vi "Send Move Command.vi"(0 "CS++Motor in":refnum<class "CS++Motor.lvclass">, 1 "Moving?":bool[](array[boolean]), 3 "MovementList In":T1(array[cluster]), 5 "error in (no error)":errorcluster, 6 "Axis Overwrite?":bool, 7 "LastPos In":dbl[](array[numeric]), 8 "SimultaneousMovement?":bool, 11 "ActPos":dbl[](array[numeric])) -> (13 "LastPos Out":dbl[](array[numeric]), 14 "CS++Motor out":refnum<class "CS++Motor.lvclass">, 17 "MovementList Out":T1(array[cluster]), 19 "error out":errorcluster)   [LabVIEW 2015, in "CS++Motor.lvlib" / "CS++Motor.lvclass"]
doc: "This VI sends the Movement Commands to the child class if necessary."
uses:
  CS++Motor.lvclass
  CSPP_Core/Classes/CS++ProcessVariables/ProcessVariable/PV.lvclass
  PV-Enum-n.ctl
  CS++Motor.lvclass/CS++Motor.ctl
  CSPP_Core/Classes/CS++ProcessVariables/ProcessVariable/PV.lvclass/PV.ctl
  CSPP_Core/Classes/CS++ProcessVariables/ProcessVariable/Write Data.vi
  CSPP_Core/Classes/CS++ProcessVariables/ProcessVariable/Write Timestamp.vi
  CSPP_Core/Classes/CS++ProcessVariables/ProcessVariable/Write Quality.vi
  CSPP_Core/Classes/CS++ProcessVariables/ProcessVariable/Write status.vi
  CSPP_Core/Classes/CS++ProcessVariables/PVConnection/PVConnection.lvclass
  CSPP_Core/Libraries/Utilities/CS++Utilities.lvlib
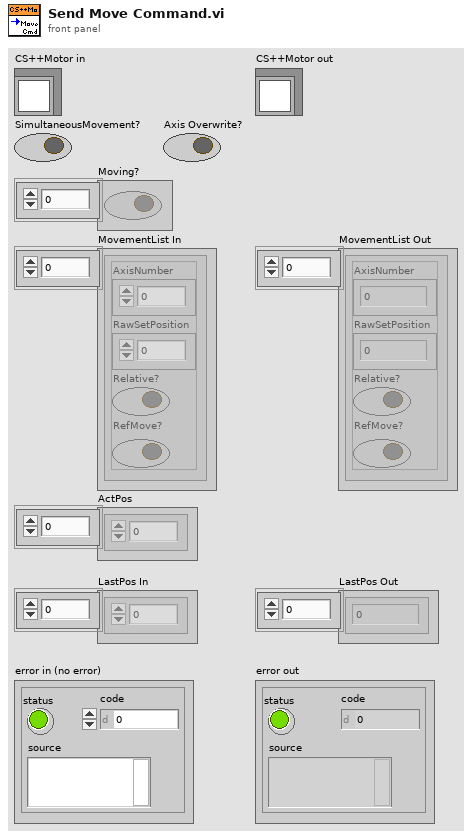
[diagram p1: front panel]
types:
  T1 = cluster{"AxisNumber":u8, "RawSetPosition":dbl, "Relative?":bool, "RefMove?":bool}[]
  T2 = typedef "CS++Motor.lvlib/CS++Motor.lvclass/PV-Enum-n.ctl" = enum16{"PhysicalName", "unit", "ActPosition", "SetPosition", "RawSetPosition", "StartVelocity", "StopVelocity", "Acceleration", "RangeMin", "RangeMax", "Scaling", "RangeRefError", "LogicalPositionArray", "NoOfCommands"}
  T3 = cluster{"AxisNumber":u8, "RawSetPosition":dbl, "Relative?":bool, "RefMove?":bool}
  T4 = cluster{"LogicalName":string, "PhysicalName":string, "unit":string, "Scaling":dbl, "StartVelocity":dbl, "StopVelocity":dbl, "Acceleration":dbl, "RangeMin":dbl, "RangeMax":dbl, "LogicalPos-Array":cluster{"LogicalPosition":string, "SetPosition":dbl}[]}[]
  T5 = cluster{"LogicalName":string, "PhysicalName":string, "unit":string, "Scaling":dbl, "StartVelocity":dbl, "StopVelocity":dbl, "Acceleration":dbl, "RangeMin":dbl, "RangeMax":dbl, "LogicalPos-Array":cluster{"LogicalPosition":string, "SetPosition":dbl}[]}
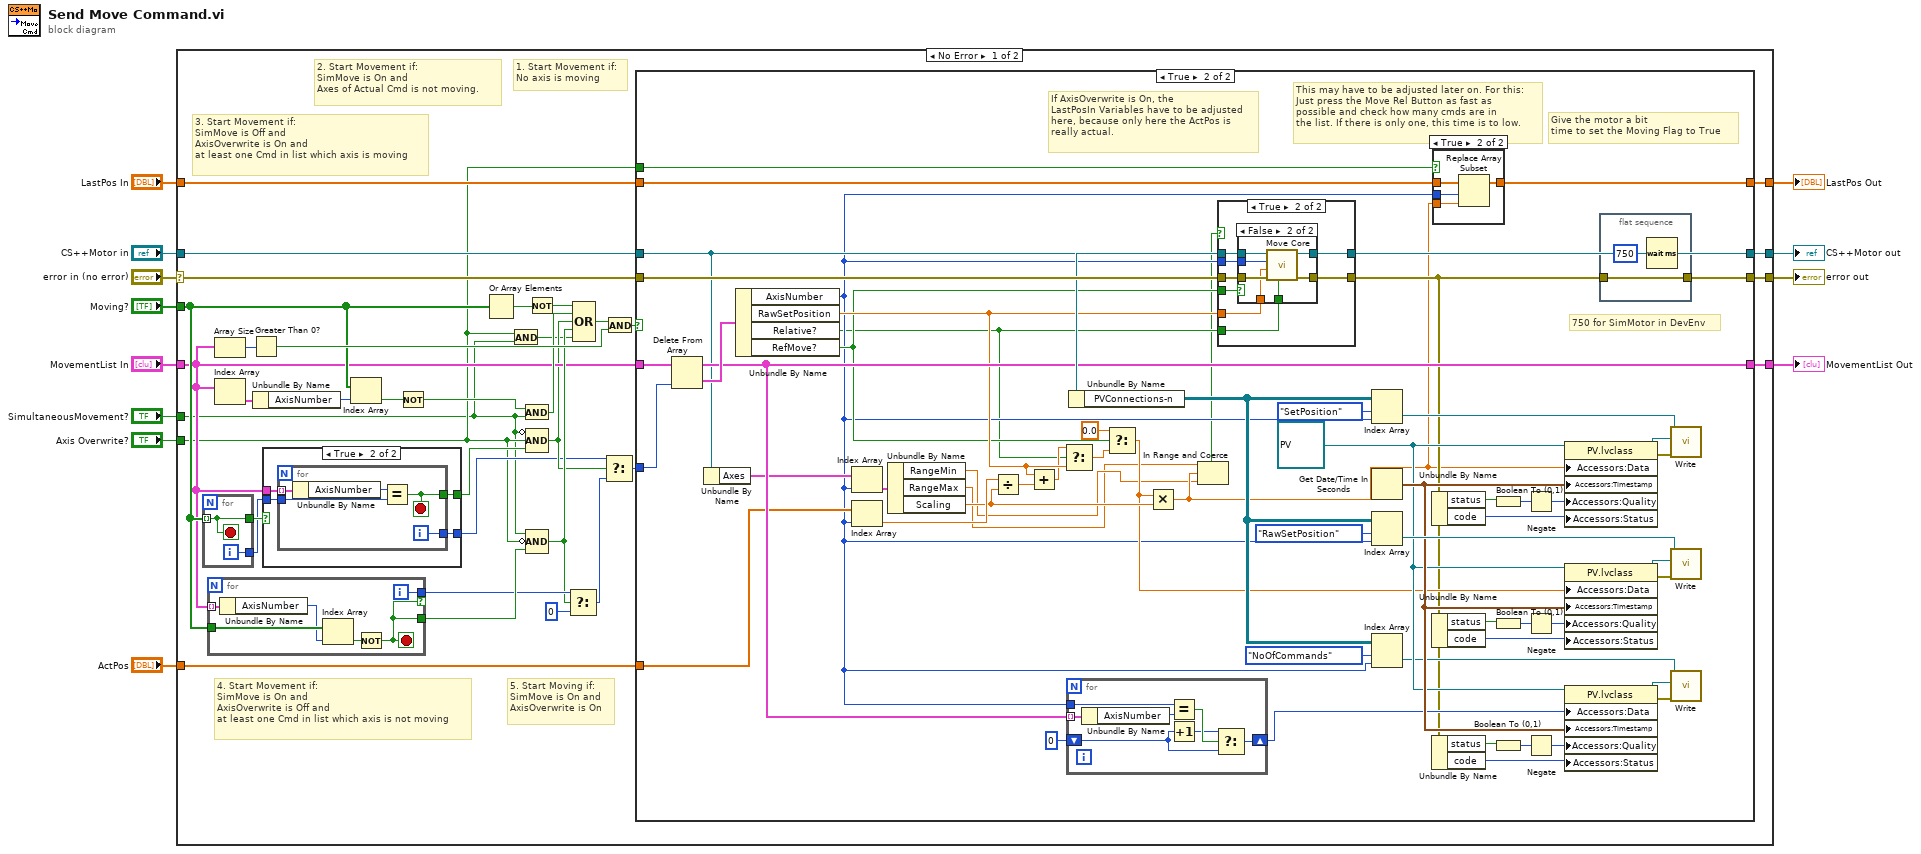
[diagram p0: block diagram]
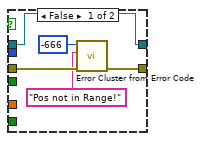
[diagram p4: hidden frame]
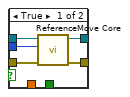
[diagram p5: hidden frame]
diagram:
  n1 = case shown="No Error" "error in (no error)" {
    selector: "error in (no error)" -> [w47 w170]
    tunnel: [w44 w170] -> w11
    tunnel: [w45 w169] -> w9
    tunnel: "CS++Motor in" -> [w40 w169]
    tunnel: "Moving?" -> [w25 _]
    tunnel: "SimultaneousMovement?" -> [w13 _]
    tunnel: "MovementList In" -> [w24 w168]
    tunnel: [w46 w168] -> w5
    tunnel: "ActPos" -> [w41 _]
    tunnel: "Axis Overwrite?" -> [w14 _]
    tunnel: "LastPos In" -> [w28 w167]
    tunnel: [w27 w167] -> w1
    frame No Error {
      # "5. Start Moving if:\nSimMove is On and\nAxisOverwrite is On"
      # "4. Start Movement if:\nSimMove is On and\nAxisOverwrite is Off and\nat least one Cmd in list which axis is not moving"
      # "3. Start Movement if:\nSimMove is Off and \nAxisOverwrite is On and\nat least one Cmd in list which axis is moving"
      # "2. Start Movement if:\nSimMove is On and\nAxes of Actual Cmd is not moving."
      # "1. Start Movement if:\nNo axis is moving"
      n2 = for {
        tunnel: w25 -> [w58] mode=indexing
        tunnel: [w58] -> w23
        tunnel: [w57] -> w17
        i -> [w57]
        stop <- w58 stop-if-true
      }
      n3 = for {
        tunnel: w24 -> [w62] mode=indexing
        tunnel: w25 -> [w64]
        tunnel: [w60] -> w31 if=w59
        tunnel: [w59] -> w33
        i -> [w60]
        stop <- w59 stop-if-true
        n4 = Unbundle By Name(w62) -> ("AxisNumber"=w63:u8)
        n5 = Index Array(array=w64, index=w63) -> (element=w61:bool)
        n6 = Not(x=w61) -> (.not. x?=w59:bool)
      }
      n7 = Array Size(array=w24) -> (size(s)=w43:i32)
      n8 = Index Array(array=w24) -> (element=w38:T3)  [unwired: 1 in]
      n9 = Greater Than 0?(x=w43) -> (x > 0?=w42:bool)
      n10 = Unbundle By Name(w38) -> ("AxisNumber"=w29:u8)
      n11 = case shown="True" w23 {
        tunnel: w24 -> [_ w51]
        tunnel: w17 -> [_ w50]
        tunnel: [_ w49] -> w18
        tunnel: [_ w48] -> w22
        frame False {
        }
        frame True {
          n12 = for {
            tunnel: w51 -> [w56] mode=indexing
            tunnel: w50 -> [w54]
            tunnel: [w53] -> w48
            tunnel: [w52] -> w49
            i -> [w52]
            stop <- w53 stop-if-true
            n13 = Unbundle By Name(w56) -> ("AxisNumber"=w55:u8)
            n14 = Equal?(x=w55, y=w54) -> (x = y?=w53:bool)
          }
        }
      }
      n15 = Index Array(array=w25, index=w29) -> (element=w37:bool)
      n16 = Not(x=w37) -> (.not. x?=w34:bool)
      n17 = Or Array Elements(Boolean array=w25) -> (logical OR=w16:bool)
      n18 = And(x=w14, y=w13) -> (x .and. y?=w15:bool)
      n19 = And(x=w34, y=w13) -> (x .and. y?=w35:bool)
      n20 = Compound Arithmetic op=AND(invert w13, w14, w22) -> (w21:bool)
      n21 = Compound Arithmetic op=AND(w13, invert w14, w33) -> (w26:bool)
      n22 = Not(x=w16) -> (.not. x?=w36:bool)
      n23 = Select(t=w31, s=w26, f=0) -> (s? t:f=w19:i32)
      n24 = Compound Arithmetic op=OR(w36, w35, w21, w26, w15) -> (w39:bool)
      n25 = Select(t=w18, s=w21, f=w19) -> (s? t:f=w20:i32)
      n26 = And(x=w39, y=w42) -> (x .and. y?=w30:bool)
      n27 = case shown="True" w30 {
        tunnel: w40 -> [w66 w94]
        tunnel: w47 -> [w67 w126]
        tunnel: w24 -> [w68 w82]
        tunnel: [w68 w97] -> w46
        tunnel: [w66 w120] -> w45
        tunnel: [w67 w80] -> w44
        tunnel: w41 -> [_ w92]
        tunnel: w20 -> [_ w78]
        tunnel: w28 -> [w65 w77]
        tunnel: [w65 w75] -> w27
        tunnel: w14 -> [_ w73]
        frame False {
        }
        frame True {
          w100 = refnum<class "PV.lvclass"> refnum ("PV")
          # "If AxisOverwrite is On, the\nLastPosIn Variables have to be adjusted\nhere, because only here the ActPos is\nreally actual."
          # "750 for SimMotor in DevEnv"
          # "This may have to be adjusted later on. For this:\nJust press the Move Rel Button as fast as\npossible and check how many cmds are in\nthe list. If there is only one, this time is to low."
          # "Give the motor a bit\ntime to set the Moving Flag to True"
          n28 = Delete From Array(array=w82, index=w78) -> (deleted portion=w127:T3, array with subset deleted=w97:T1)  [unwired: 1 in]
          n29 = Unbundle By Name(w94) -> ("Axes"=w93:T4)
          n30 = Unbundle By Name(w127) -> ("AxisNumber"=w76:u8, "RawSetPosition"=w88:dbl, "Relative?"=w74:bool, "RefMove?"=w81:bool)
          n31 = Index Array(array=w93, index=w76) -> (element=w91:T5)
          n32 = Index Array(array=w92, index=w76) -> (element=w90:dbl)
          n33 = Unbundle By Name(w91) -> ("RangeMin"=w70:dbl, "RangeMax"=w69:dbl, "Scaling"=w86:dbl)
          n34 = Divide(x=w90, y=w86) -> (x/y=w89:dbl)
          n35 = Add(x=w88, y=w89) -> (x+y=w87:dbl)
          n36 = Select(t=w87, s=w74, f=w88) -> (s? t:f=w84:dbl)
          n37 = for {
            tunnel: w97 -> [w166] mode=indexing
            tunnel: w76 -> [w164]
            shift-right: [w162] -> w95
            shift-left: 0 -> [w160]
            n38 = Unbundle By Name(w166) -> ("AxisNumber"=w165:u8)
            n39 = Equal?(x=w164, y=w165) -> (x = y?=w163:bool)
            n40 = Increment(x=w160) -> (x+1=w161:i32)
            n41 = Select(t=w161, s=w163, f=w160) -> (s? t:f=w162:i32)
          }
          n42 = Select(t=0.0, s=w81, f=w84) -> (s? t:f=w85:dbl)
          n43 = Multiply(x=w85, y=w86) -> (x*y=w72:dbl)
          n44 = In Range and Coerce(upper limit=w69, x=w72, lower limit=w70) -> (In Range?=w71:bool)  [unwired: 1 out]
          n45 = case shown="True" w71 {
            tunnel: w126 -> [w131 w140]
            tunnel: [w130 w139] -> w120
            tunnel: w94 -> [w130 w138]
            tunnel: w88 -> [_ w137]
            tunnel: w81 -> [_ w136]
            tunnel: [w132 w135] -> w79
            tunnel: w76 -> [_ w134]
            tunnel: w74 -> [_ w133]
            frame False {
              n46 = call "Error Cluster from Error Code.vi"("Error In"=w131, "Error Message (\"\")"="Pos not in Range!" ("Error Message (\"\")"), "Error Code (0)"=-666) -> ("Error Out"=w132:errorcluster)  [unwired: 8 in]
            }
            frame True {
              n47 = case shown="False" w136 {
                tunnel: w138 -> [w145 w152]
                tunnel: [w144 w151] -> w139
                tunnel: w140 -> [w143 w150]
                tunnel: [w141 w146] -> w135
                tunnel: w137 -> [_ w149]
                tunnel: w133 -> [_ w148]
                tunnel: w134 -> [w142 w147]
                frame True {
                  n48 = call-dynamic "ReferenceMove Core.vi"("error in (no error)"=w143, "AxisNumber"=w142, "CS++Motor in"=w145) -> ("error out"=w141:errorcluster, "CS++Motor out"=w144:refnum<class "CS++Motor.lvclass">)  [unwired: 7 in]
                }
                frame False {
                  n49 = call-dynamic "Move Core.vi"("Relative?"=w148, "error in (no error)"=w150, "Raw-Position"=w149, "AxisNumber"=w147, "CS++Motor in"=w152) -> ("error out"=w146:errorcluster, "CS++Motor out"=w151:refnum<class "CS++Motor.lvclass">)  [unwired: 5 in]
                }
              }
            }
          }
          n50 = Unbundle By Name(w120) -> ("PVConnections-n"=w98:refnum<class "PVConnection.lvclass">[][])
          n51 = Index Array(array=w98, index (row)=PV-Enum-n."SetPosition" ("PV-Enum-n"), index (col)=w76) -> (element=w121:refnum<class "PVConnection.lvclass">)
          n52 = Get Date/Time In Seconds() -> (seconds since 1Jan1904=w101:timestamp)
          n53 = Index Array(array=w98, index (row)=PV-Enum-n."RawSetPosition" ("PV-Enum-n"), index (col)=w76) -> (element=w115:refnum<class "PVConnection.lvclass">)
          n54 = Index Array(array=w98, index (row)=PV-Enum-n."NoOfCommands" ("PV-Enum-n"), index (col)=w76) -> (element=w99:refnum<class "PVConnection.lvclass">)
          n55 = Unbundle By Name(w79) -> ("status"=w124:bool, "code"=w119:i32)
          n56 = Unbundle By Name(w79) -> ("status"=w112:bool, "code"=w116:i32)
          n57 = Unbundle By Name(w79) -> ("status"=w106:bool, "code"=w103:i32)
          n58 = case shown="True" w73 {
            tunnel: w77 -> [w153 w157]
            tunnel: w76 -> [_ w156]
            tunnel: [w153 w155] -> w75
            tunnel: w72 -> [_ w154]
            frame False {
            }
            frame True {
              n59 = Replace Array Subset(array=w157, new element=w154, index=w156) -> (w155:dbl[])
            }
          }
          n60 = Boolean To (0,1)(Boolean=w124) -> (0, 1=w118:i16)
          n61 = Boolean To (0,1)(Boolean=w112) -> (0, 1=w117:i16)
          n62 = Boolean To (0,1)(Boolean=w106) -> (0, 1=w102:i16)
          n63 = Negate(x=w118) -> (-x=w125:i16)
          n64 = Negate(x=w117) -> (-x=w111:i16)
          n65 = Negate(x=w102) -> (-x=w107:i16)
          n66 = property class="PV.lvclass"(reference=w100, "Accessors:Data"=w72, "Accessors:Timestamp"=w101, "Accessors:Quality"=w125, "Accessors:Status"=w119) -> (reference out=w123:refnum<class "PV.lvclass">, error out=w122:errorcluster)  [unwired: 1 in]
          n67 = property class="PV.lvclass"(reference=w100, "Accessors:Data"=w85, "Accessors:Timestamp"=w101, "Accessors:Quality"=w111, "Accessors:Status"=w116) -> (reference out=w113:refnum<class "PV.lvclass">, error out=w114:errorcluster)  [unwired: 1 in]
          n68 = property class="PV.lvclass"(reference=w100, "Accessors:Data"=w95, "Accessors:Timestamp"=w101, "Accessors:Quality"=w107, "Accessors:Status"=w103) -> (reference out=w105:refnum<class "PV.lvclass">, error out=w104:errorcluster)  [unwired: 1 in]
          n69 = flat-sequence {
            tunnel: [w159] -> w80
            tunnel: w79 -> [w159]
            frame #0 {
              n70 = Wait (ms)(milliseconds to wait=u32 750) -> ()  [unwired: 1 out]
            }
          }
          n71 = call "Write.vi"("error in (no error)"=w122, "PV"=w123, "PVConnection in"=w121) -> ()  [unwired: 7 in, 2 out]
          n72 = call "Write.vi"("error in (no error)"=w114, "PV"=w113, "PVConnection in"=w115) -> ()  [unwired: 7 in, 2 out]
          n73 = call "Write.vi"("error in (no error)"=w104, "PV"=w105, "PVConnection in"=w99) -> ()  [unwired: 7 in, 2 out]
        }
      }
    }
    frame Error {
    }
  }
  "error out" <- w11
  "CS++Motor out" <- w9
  "MovementList Out" <- w5
  "LastPos Out" <- w1
